vi "TimeLmtDialog.vi"(8 "颜色盒":u32(colorbox), 9 "time(s)":i32=5, 10 "Infoin":string="在这里填写显示的信息内容", 11 "title":string="提示信息") -> ()   [LabVIEW 2016, in "斯坦道总磷总氮.lvlib"]
uses:
  <vilib>/Utility/miscctls.llb/LVPointTypeDef.ctl
panel:
  in  "ok":bool
  out "info":string
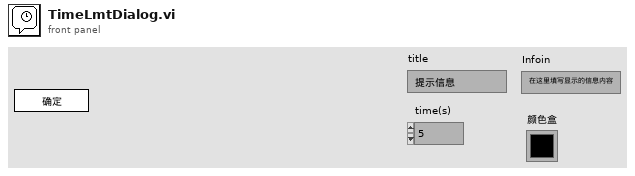
[diagram p1: front panel]
types:
  T1 = typedef "LVPointTypeDef.ctl" = cluster{"Horizontal":i16, "Vertical":i16}
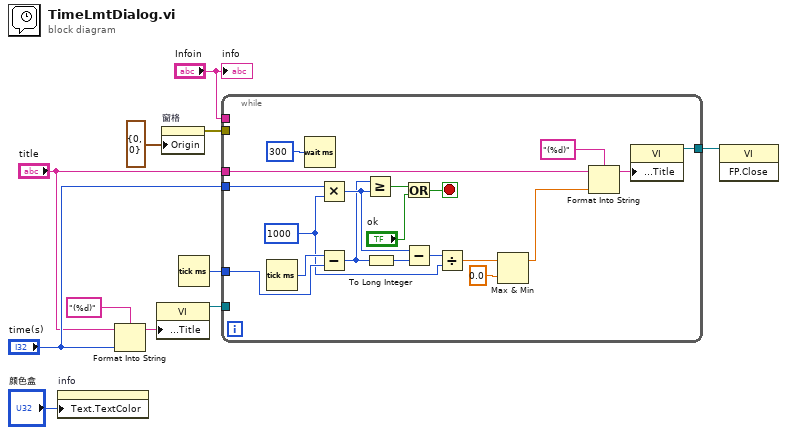
[diagram p0: block diagram]
diagram:
  n1 = property on="info" class="Str"("Text.TextColor"="颜色盒") -> ()  [unwired: 2 in, 2 out]
  n2 = Format Into String(format string="(%d)" ("格式字符串"), initial string="title", "time(s)") -> (resulting string=w7:string)  [unwired: 1 in, 1 out]
  n3 = property class="VI"("Front Panel.Title"=w7) -> (reference out=w10:refnum<vi>)  [unwired: 2 in, 1 out]
  n4 = property on="窗格" class="Pane"("Origin"=T1 {"Horizontal"=0, "Vertical"=0} ("原点")) -> (error out=w1:errorcluster)  [unwired: 2 in, 1 out]
  n5 = Tick Count (ms)() -> (millisecond timer value=w5:u32)
  n6 = while {
    tunnel: "Infoin" -> [_]
    tunnel: "time(s)" -> [w27]
    tunnel: w10 -> [_]
    tunnel: "title" -> [w19]
    tunnel: w5 -> [w28]
    tunnel: [w12] -> w4
    tunnel: w1 -> [_]
    stop <- w24 stop-if-true
    w20 = 1000 ("y")
    n7 = Tick Count (ms)() -> (millisecond timer value=w29:u32)
    n8 = Wait (ms)(milliseconds to wait=u32 300 ("等待时间（毫秒）")) -> ()  [unwired: 1 out]
    n9 = Multiply(x=w27, y=w20) -> (x*y=w23:i32)
    n10 = Subtract(x=w29, y=w28) -> (x-y=w22:u32)
    n11 = Greater Or Equal?(x=w22, y=w23) -> (x >= y?=w25:bool)
    n12 = To Long Integer(number=w22) -> (32bit integer=w13:i32)
    n13 = Or(x=w25, y="ok") -> (x .or. y?=w24:bool)
    n14 = Subtract(x=w23, y=w13) -> (x-y=w21:i32)
    n15 = Divide(x=w21, y=w20) -> (x/y=w16:dbl)
    n16 = Max & Min(x=w16, y=0.0) -> (max(x,y)=w14:dbl)  [unwired: 1 out]
    n17 = Format Into String(format string="(%d)" ("格式字符串"), initial string=w19, w14) -> (resulting string=w17:string)  [unwired: 1 in, 1 out]
    n18 = property class="VI"("Front Panel.Title"=w17) -> (reference out=w12:refnum<vi>)  [unwired: 2 in, 1 out]
  }
  n19 = invoke class="VI" method="FP.Close"(reference=w4) -> ()  [unwired: 2 in, 3 out]
  "info" <- "Infoin"
